vi "Send Voltage.vi"(8 "error in":errorcluster, 11 "4322 in":refnum<class "4322.lvclass">) -> (0 "error out":errorcluster, 3 "4322 out":refnum<class "4322.lvclass">)   [LabVIEW 2019, in "4322.lvlib" / "4322.lvclass"]
uses:
  Library/4322.lvclass
  C:/Users/Public/Documents/Development/builds/Instruments/Analog-Output.lvlibp/Library/Analog-Output.lvclass
  Library/4322.lvclass/4322.ctl
  <vilib>/DAQmx/write.llb/DAQmx Write (Analog 1D DBL NChan 1Samp).vi
  Accessors/Read Local Resource.vi
  Accessors/Write Local Resource.vi
  builds/Instruments/Analog-Output.lvlibp/Accessors/Read All Voltages.vi
  <vilib>/DAQmx/miscellaneous.llb/DAQmx Fill In Error Info.vi
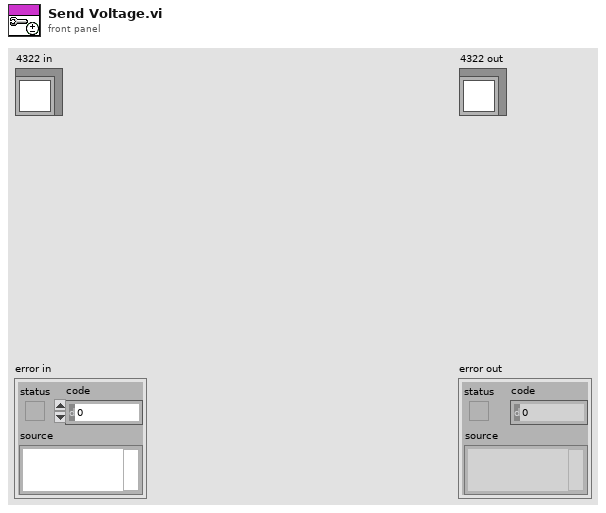
[diagram p1: front panel]
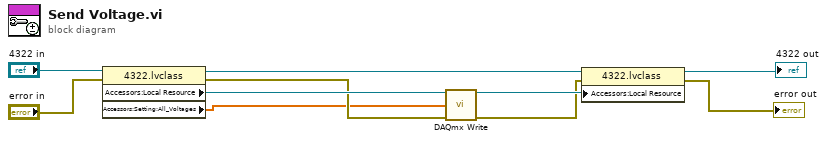
[diagram p0: block diagram]
diagram:
  n1 = property class="4322.lvclass"(reference="4322 in", error in="error in") -> (reference out=w7:refnum<class "4322.lvclass">, error out=w5:errorcluster, "Accessors:Local Resource"=w10:refnum<k21>, "Accessors:Setting:All_Voltages"=w1:dbl[])
  n2 = call-poly <vilib>:"DAQmx Write.vi"("task/channels in"=w10, "data"=w1, "error in"=w5) -> ("task out"=w9:refnum<k21>, "error out"=w4:errorcluster)  [unwired: 10 in, 1 out]
  n3 = property class="4322.lvclass"(reference=w7, error in=w4, "Accessors:Local Resource"=w9) -> (reference out=→"4322 out":refnum<class "4322.lvclass">, error out=→"error out":errorcluster)
